vi "DrivePID.vi"(7 "Compensate":bool, 9 "SetpointLeft":dbl format="%.2f", 11 "SetpointRight":dbl format="%.2f") -> (15 "Done":bool)   [LabVIEW 2014]
uses:
  <vilib>/addons/control/pid/pid.llb/PID (DBL).vi
  <vilib>/Rock Robotics/WPI/RobotDrive/WPI_RobotDriveGetSetRefNum.vi
  <vilib>/addons/control/pid/NI_PID_pid.lvlib
panel:
  in  "RightDriveRefNum":string="My Encoder RefNum"
  in  "LeftDriveRefNum":string="My Encoder RefNum"
  in  "PID gains for motor gain":T1={"proportional gain (Kc)"=1.0, "integral time (Ti, min)"=0.01, "derivative time (Td, min)"=0.0} {"derivative time (Td, min)" format="%.3f"; "integral time (Ti, min)" format="%.3f"; "proportional gain (Kc)" format="%.3f"}
  in  "PID gains Right":T1={"proportional gain (Kc)"=0.5, "integral time (Ti, min)"=1e-05, "derivative time (Td, min)"=0.001} {"derivative time (Td, min)" format="%.3f"; "integral time (Ti, min)" format="%.7f"; "proportional gain (Kc)" format="%.3f"}
  out "Right Chart":dbl(graph)
  out "Left Chart":dbl(graph)
  in  "PID gains Left":T1={"proportional gain (Kc)"=0.5, "integral time (Ti, min)"=1e-05, "derivative time (Td, min)"=0.001} {"derivative time (Td, min)" format="%.3f"; "integral time (Ti, min)" format="%.7f"; "proportional gain (Kc)" format="%.3f"}
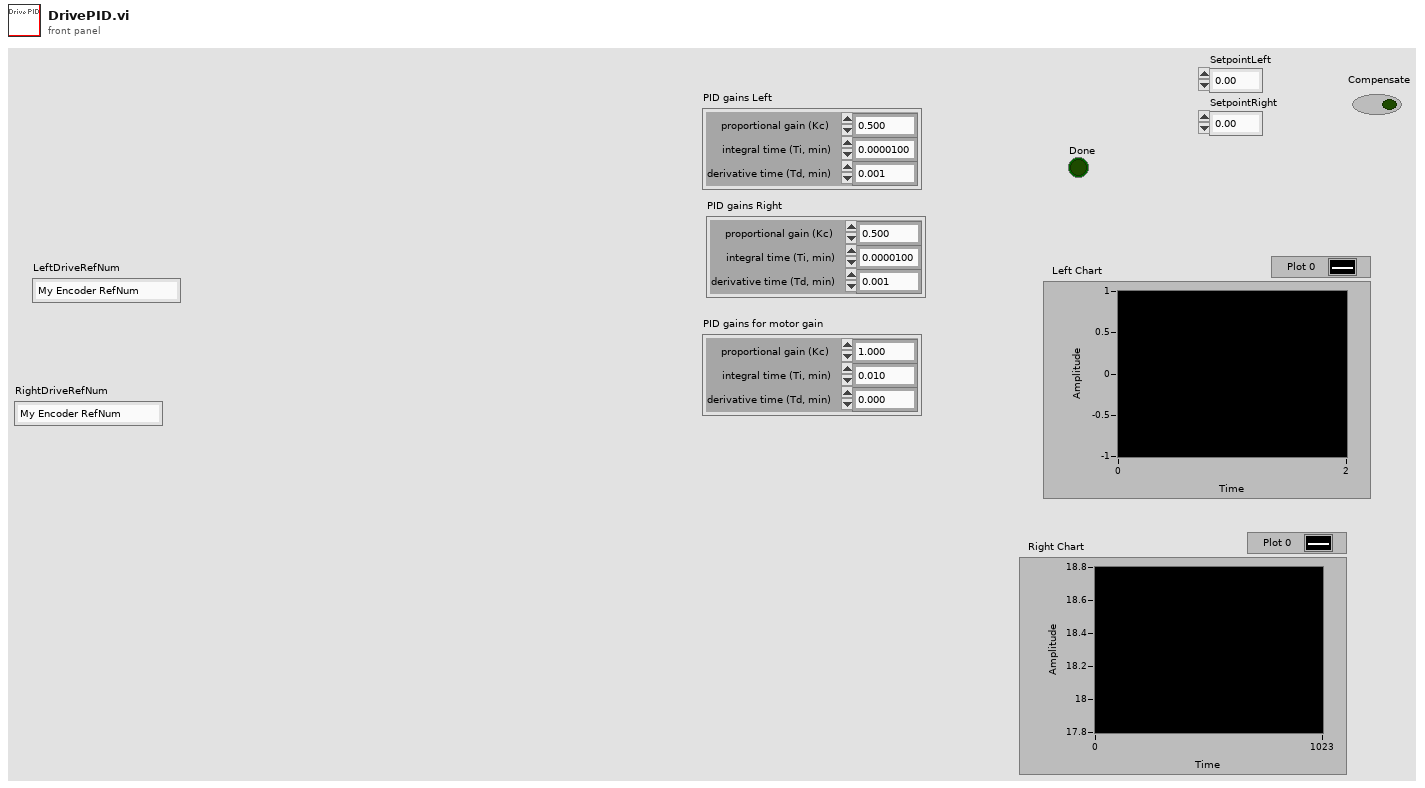
[diagram p1: front panel]
types:
  T1 = cluster{"proportional gain (Kc)":dbl, "integral time (Ti, min)":dbl, "derivative time (Td, min)":dbl}
  T2 = typedef "WPI_EncoderDevRef.ctl" = cluster{"DevStatus":errorcluster, "EncoderIndex":T3, "CounterIndex":T4, "DistancePerCount":dbl, "Decoding Type":T5}
  T3 = typedef "FPGA_EncoderIdx.ctl" = enum8{"Enc 0", "Enc 1", "Enc 2", "Enc 3", "Enc 4", "Enc 5", "Enc 6", "Enc 7", "Invalid"}
  T4 = typedef "FPGA_CounterCtrSystemIndex.ctl" = enum8{"Ctr 0", "Ctr 1", "Ctr 2", "Ctr 3", "Ctr 4", "Ctr 5", "Ctr 6", "Ctr 7", "Invalid"}
  T5 = typedef "WPI_EncoderType.ctl" = enum16{"1x", "2x", "4x"}
  T6 = typedef "WPI_RobotDriveDevRef.ctl" = cluster{"DevStatus":errorcluster, "Motors[]":T7[], "Square Inputs":bool, "Max Output":dbl}
  T7 = typedef "WPI_MotorControlDeviceRef.ctl" = cluster{"DeviceStatus":errorcluster, "Type":T8, "PWM":cluster{"Controller":T9, "PWM Channel":T10, "DeadBand":T11}, "CAN":cluster{"Device Number":u8, "Control Mode":T12, "Semaphore":T13, "Max Vout":dbl, "TalonSRX Control Mode":T14}, "Invert":bool, "TransformRef":T15, "InvTransformRef":T15}
  T8 = typedef "WPI_MotorControlType.ctl" = enum16{"PWM", "CAN", "CANTalonSRX"}
  T9 = typedef "FPGA_TypedefDigitalModule.ctl" = enum16{"Controller 1"}
  T10 = typedef "FPGA_DIOPWMChannel.ctl" = enum8{"PWM 0", "PWM 1", "PWM 2", "PWM 3", "PWM 4", "PWM 5", "PWM 6", "PWM 7", "PWM 8", "PWM 9", "PWM MXP 0", "PWM MXP 1", "PWM MXP 2", "PWM MXP 3", "PWM MXP 4", "PWM MXP 5", "PWM MXP 6", "PWM MXP 7", "PWM MXP 8", "PWM MXP 9", "Invalid"}
  T11 = typedef "WPI_PWMDeadband.ctl" = cluster{"Name":string, "maxPositivePwm":i32, "minPositivePwm":i32, "centerPwm":i32, "maxNegativePwm":i32, "minNegativePwm":i32, "angularRange":u16}
  T12 = typedef "WPI_CANJaguar_ControlMode.ctl" = enum8{"Percent VBus", "Current", "Speed", "Position", "Voltage"}
  T13 = typedef "Semaphore RefNum" = refnum<k1>
  T14 = typedef "WPI_CANTalonSRX_APIControlMode.ctl" = enum8{"Percent VBus", "Speed", "Position", "Slave", "Unchanged / Invalid"}
  T15 = typedef "WPI_PWMTransform_ConPane.ctl" = refnum<vi>
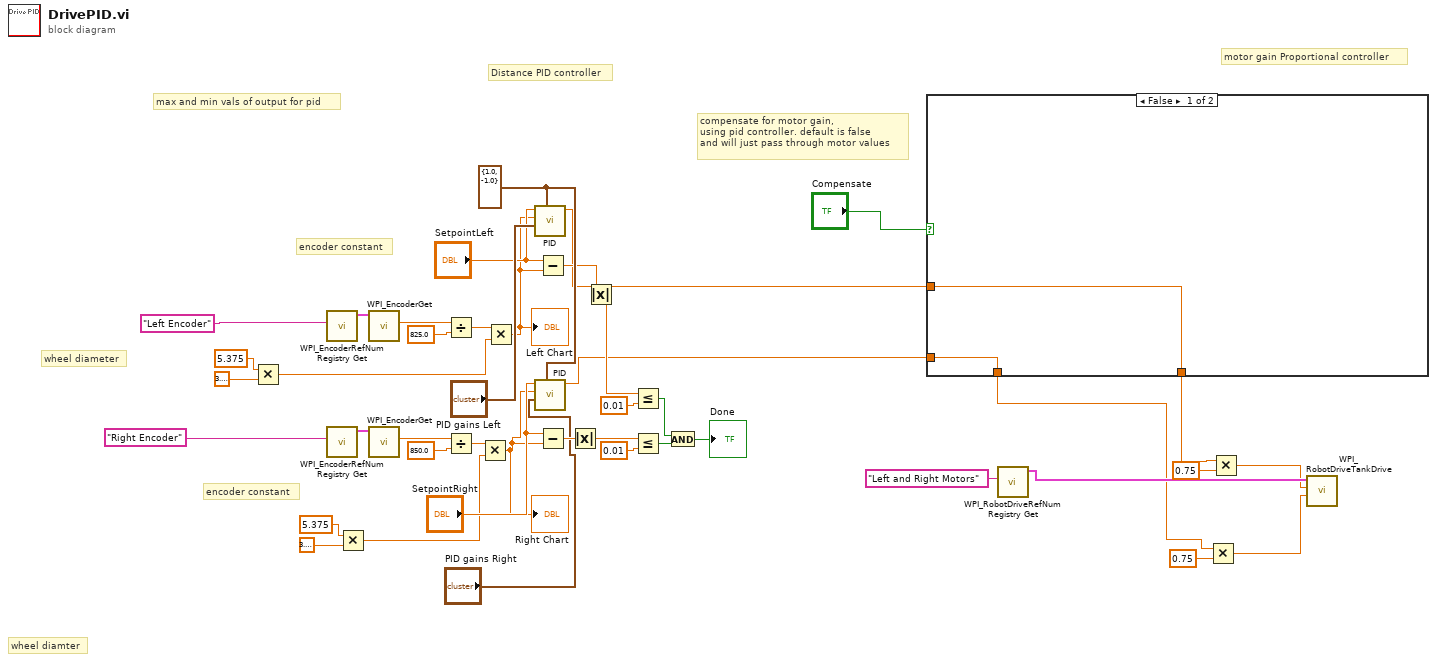
[diagram p0: block diagram]
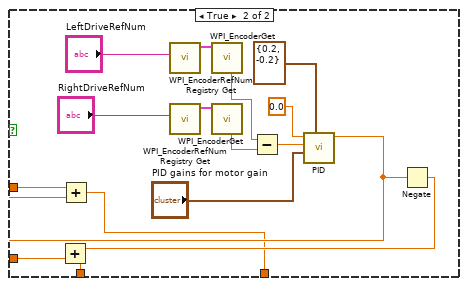
[diagram p2: hidden frame]
diagram:
  w40 = cluster{"output high":dbl, "output low":dbl} {"output high"=1.0, "output low"=-1.0} ("output range")
  # "compensate for motor gain,\nusing pid controller. default is false\nand will just pass through motor values"
  # "max and min vals of output for pid"
  # "encoder constant"
  # "encoder constant"
  # "wheel diamter"
  # "wheel diameter"
  # "motor gain Proportional controller"
  # "Distance PID controller"
  n1 = Multiply(x=5.375, y=3.141592653589793) -> (x*y=w19:dbl)
  n2 = call <vilib>:"WPI_EncoderRefNum Registry Get.vi"("refnum name"="Left Encoder") -> ("EncoderDevRef"=w43:T2)  [unwired: 9 in, 1 out]
  n3 = call <vilib>:"WPI_EncoderRefNum Registry Get.vi"("refnum name"="Right Encoder") -> ("EncoderDevRef"=w37:T2)  [unwired: 9 in, 1 out]
  n4 = Multiply(x=5.375, y=3.141592653589793) -> (x*y=w16:dbl)
  n5 = call <vilib>:"WPI_EncoderGet.vi"("EncoderDevRef"=w43) -> ("Distance"=w24:dbl)  [unwired: 5 in, 5 out]
  n6 = call <vilib>:"WPI_EncoderGet.vi"("EncoderDevRef"=w37) -> ("Distance"=w23:dbl)  [unwired: 5 in, 5 out]
  n7 = Divide(x=w24, y=825.0) -> (x/y=w20:dbl)
  n8 = Divide(x=w23, y=850.0) -> (x/y=w17:dbl)
  n9 = Multiply(x=w17, y=w16) -> (x*y=w14:dbl)
  "Right Chart" <- w14
  n10 = Multiply(x=w20, y=w19) -> (x*y=w18:dbl)
  "Left Chart" <- w18
  n11 = call-poly <vilib>:"PID.vi"("output range"=w40, "PID gains"="PID gains Left", "process variable"=w18, "setpoint"="SetpointLeft") -> ("output"=w12:dbl)  [unwired: 6 in, 1 out]
  n12 = call-poly <vilib>:"PID.vi"("output range"=w40, "PID gains"="PID gains Right", "process variable"=w14, "setpoint"="SetpointRight") -> ("output"=w13:dbl)  [unwired: 6 in, 1 out]
  n13 = Subtract(x="SetpointLeft", y=w18) -> (x-y=w38:dbl)
  n14 = Subtract(x="SetpointRight", y=w14) -> (x-y=w31:dbl)
  n15 = Absolute Value(x=w31) -> (abs(x)=w21:dbl)
  n16 = Absolute Value(x=w38) -> (abs(x)=w22:dbl)
  n17 = Less Or Equal?(x=w22, y=0.01) -> (x <= y?=w34:bool)
  n18 = Less Or Equal?(x=w21, y=0.01) -> (x <= y?=w35:bool)
  n19 = And(x=w34, y=w35) -> (x .and. y?=→"Done":bool)
  n20 = case shown="False" "Compensate" {
    tunnel: w13 -> [w44 w51]
    tunnel: [w44 w49] -> w5
    tunnel: w12 -> [w45 w48]
    tunnel: [w45 w46] -> w6
    frame False {
    }
    frame True {
      n21 = call <vilib>:"WPI_EncoderRefNum Registry Get.vi"("refnum name"="LeftDriveRefNum") -> ("EncoderDevRef"=w60:T2)  [unwired: 9 in, 1 out]
      n22 = call <vilib>:"WPI_EncoderRefNum Registry Get.vi"("refnum name"="RightDriveRefNum") -> ("EncoderDevRef"=w57:T2)  [unwired: 9 in, 1 out]
      n23 = call <vilib>:"WPI_EncoderGet.vi"("EncoderDevRef"=w60) -> ("Rate"=w55:dbl)  [unwired: 5 in, 5 out]
      n24 = call <vilib>:"WPI_EncoderGet.vi"("EncoderDevRef"=w57) -> ("Rate"=w54:dbl)  [unwired: 5 in, 5 out]
      n25 = Subtract(x=w55, y=w54) -> (x-y=w52:dbl)
      n26 = call-poly <vilib>:"PID.vi"("output range"=cluster{"output high":dbl, "output low":dbl} {"output high"=0.2, "output low"=-0.2}, "PID gains"="PID gains for motor gain", "process variable"=w52, "setpoint"=0.0) -> ("output"=w47:dbl)  [unwired: 6 in, 1 out]
      n27 = Add(x=w48, y=w47) -> (x+y=w46:dbl)
      n28 = Negate(x=w47) -> (-x=w50:dbl)
      n29 = Add(x=w50, y=w51) -> (x+y=w49:dbl)
    }
  }
  n30 = call <vilib>:"WPI_RobotDriveRefNum Registry Get.vi"("refnum name"="Left and Right Motors") -> ("RobotDriveDevRef"=w7:T6)  [unwired: 9 in, 1 out]
  n31 = Multiply(x=w5, y=0.75) -> (x*y=w1:dbl)
  n32 = Multiply(x=w6, y=0.75) -> (x*y=w2:dbl)
  n33 = call <vilib>:"WPI_RobotDriveTankDrive.vi"("Right axis value"=w1, "Left axis value"=w2, "RobotDriveDevRef"=w7) -> ()  [unwired: 6 in, 3 out]
